vi "EmptyExperiment.vi"() -> ()   [LabVIEW 2017]
uses:
  Expose/Labview/Parameters/ExposeParameterBindingType.ctl
panel:
  in  "Call MyMethod":bool
  in  "ExampleStruct":cluster{"Val":dbl, "String":string}
  in  "ExampleValue":dbl
  in  "ExampleButton":bool
  out "IsBusy":bool=TRUE
  out "ExpID":string="Exp967f258c607eed45caf40f4c3101458dC" caption="Exp. ID (Debug)"
  out "ExampleGraph":dbl[](graph)
  # "The code file (.m) is under the same name as the labview file"
  # "Bound controls pannel: All controls in this pannel will\nbe bidirectionally bound to the matlab class. \n(Flat sequence step 2)"
  # "Bound indicatios pannel: All controls in this pannel will\nbe updated FROM matlab only\n(Flat sequence step 2)"
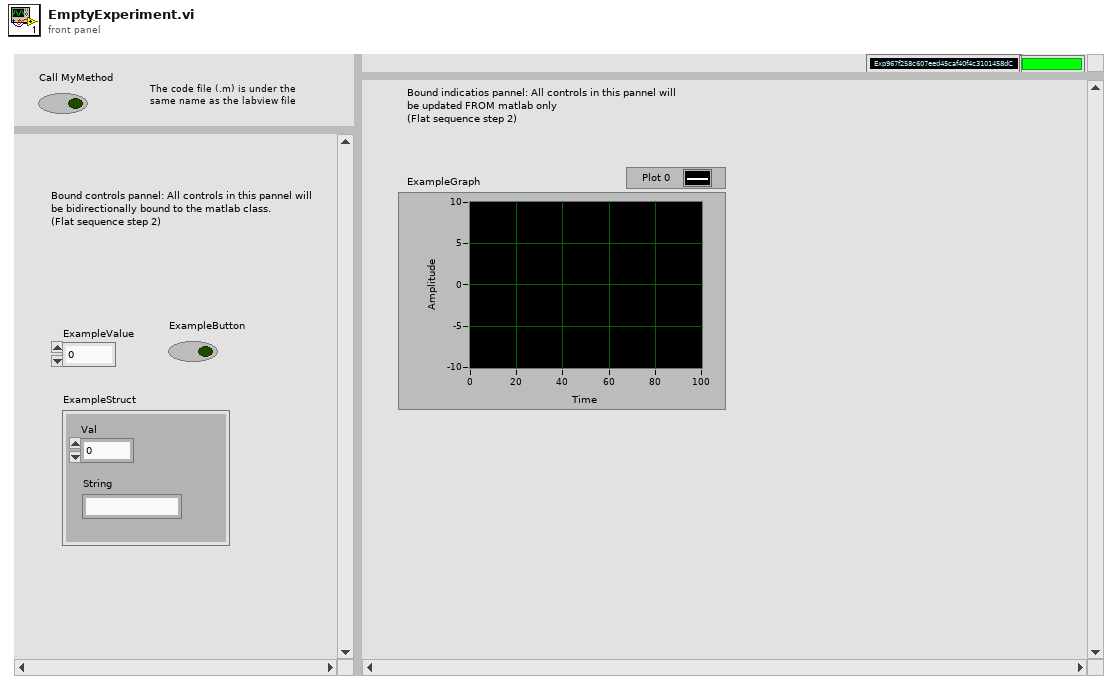
[diagram p1: front panel]
types:
  T1 = typedef "ExposeParameterBindingType.ctl" = enum16{"ToRemote", "FromRemote", "Bidrectional"}
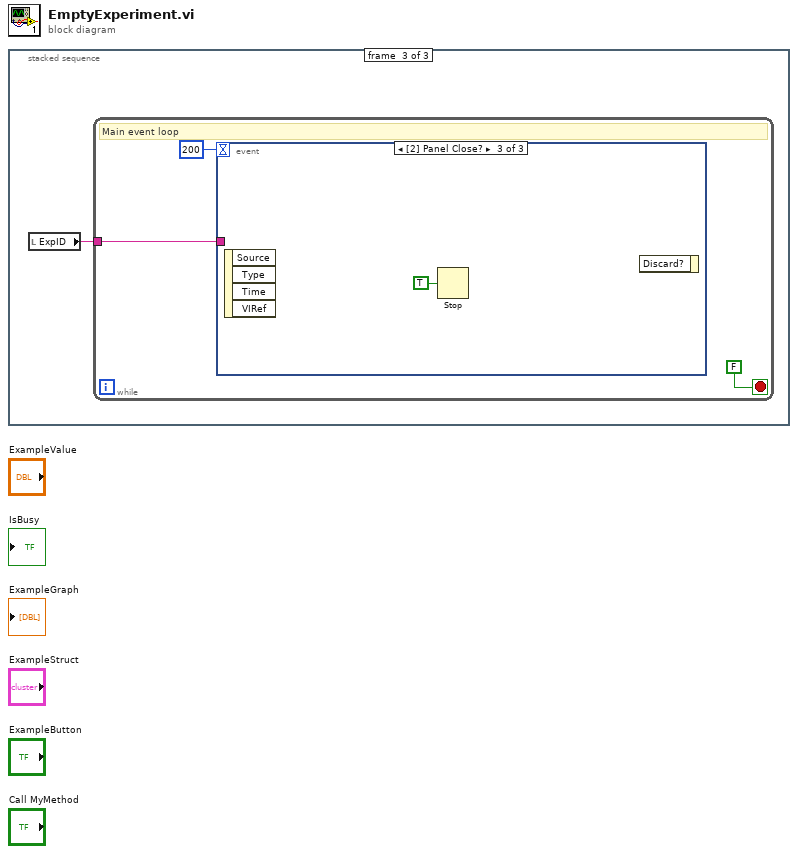
[diagram p0: block diagram]
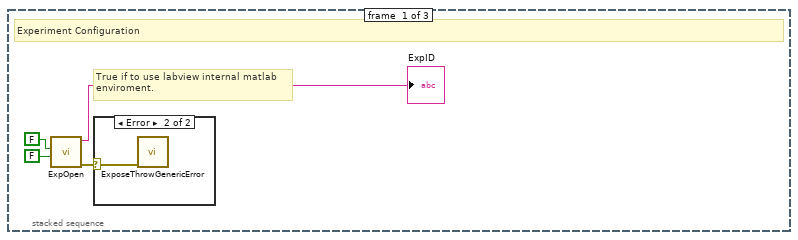
[diagram p2: hidden frame]
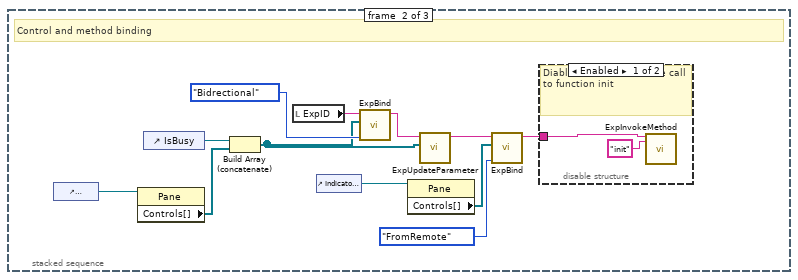
[diagram p4: hidden frame]
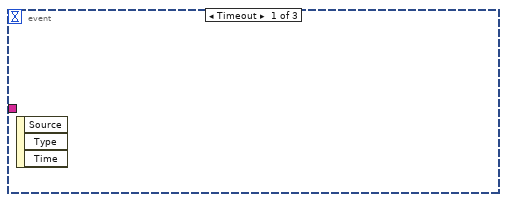
[diagram p6: hidden frame]
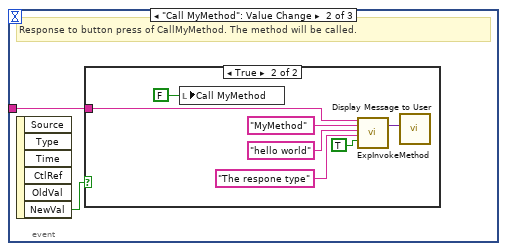
[diagram p7: hidden frame]
diagram:
  n1 = stacked-sequence {
    frame #0 {
      # "True if to use labview internal matlab\nenviroment."
      # "Experiment Configuration"
      n2 = call "ExpOpen.vi"("Do Expose Logging"=FALSE, "Requires Matlab Enviroment"=FALSE) -> ("error out"=w2:errorcluster, "ExpID"=→"ExpID":string)  [unwired: 7 in, 1 out]
      n3 = case shown="Error" w2 {
        selector: w2 -> [_ w5]
        frame No Error {
        }
        frame Error {
          n4 = call "ExposeThrowGenericError.vi"("error in (no error)"=w5) -> ()  [unwired: 10 in, 1 out]
        }
      }
    }
    frame #1 {
      # "Control and method binding"
      n5 = control-ref of="ControlsPane"() -> (w9:refnum<vi>)
      n6 = property class="Pane"(reference=w9) -> ("Controls[]"=w16:refnum<vi>[])  [unwired: 1 in, 2 out]
      n7 = control-ref of="IsBusy"() -> (w17:refnum<vi>)
      n8 = Build Array (concatenate)(w17, w16) -> (w8:refnum<vi>[])
      n9 = local read "ExpID"() -> (w15:string)
      n10 = control-ref of="Indicator Pane"() -> (w11:refnum<vi>)
      n11 = call "ExpBind.vi"("Binding Type"=ExposeParameterBindingType."Bidrectional", "Value"=w8, "ExpID"=w15) -> ("ExpID out"=w7:string)  [unwired: 7 in, 1 out]
      n12 = property class="Pane"(reference=w11) -> ("Controls[]"=w10:refnum<vi>[])  [unwired: 1 in, 2 out]
      n13 = call "ExpUpdateParameter.vi"("Variant"=w8, "ExpID"=w7) -> ("ExpID out"=w6:string)  [unwired: 8 in, 1 out]
      n14 = call "ExpBind.vi"("Binding Type"=ExposeParameterBindingType."FromRemote", "Value"=w10, "ExpID"=w6) -> ("ExpID out"=w13:string)  [unwired: 7 in, 1 out]
      n15 = disable-structure shown="Enabled" {
        disable-tunnel: w13 -> [w19 _]
        frame Enabled {
          # "Diable this to remove the call to function init"
          n16 = call "ExpInvokeMethod.vi"("ExpID"=w19, "Method Name"="init") -> ()  [unwired: 15 in, 3 out]
        }
        frame Disabled {
        }
      }
    }
    frame #2 {
      n17 = local read "ExpID"() -> (w20:string)
      n18 = while {
        tunnel: w20 -> [w21]
        stop <- FALSE stop-if-true
        # "Main event loop"
        n19 = event shown="[2] Panel Close?" {
          selector: _ -> [_ _ _]
          dyn-events: _ -> [_ _ _]
          timeout: 200 -> [_ _ _]
          tunnel: w21 -> [_ w24 _]
          event Timeout {
            n20 = event-data() -> ()  [unwired: 1 in, 3 out]
          }
          event "Call MyMethod": Value Change {
            # "Response to button press of CallMyMethod. The method will be called."
            n21 = event-data() -> ("NewVal"=w25:bool)  [unwired: 1 in, 5 out]
            n22 = case shown="True" w25 {
              tunnel: w24 -> [_ w32]
              frame False {
              }
              frame True {
                n23 = local write "Call MyMethod"(FALSE ("Call MyMethod")) -> ()
                n24 = call "ExpInvokeMethod.vi"("ExpID"=w32, "Method Name"="MyMethod", "Argument(s)"="hello world", "Rsp. Type (or value to update)"="The respone type", "Require Response"=TRUE) -> ("Response"=w27:variant)  [unwired: 12 in, 2 out]
                n25 = call "Display Message to User"("Message"=w27) -> ()  [unwired: 9 in, 2 out]
              }
            }
          }
          event Panel Close? {
            n26 = event-data() -> ()  [unwired: 1 in, 4 out]
            n27 = Stop(stop? (T)=TRUE) -> ()
            n28 = event-data() -> ()  [unwired: 2 in, 1 out]
          }
        }
      }
    }
  }
